vi "Safety systems data.vi"(7 "Arm System Status":bool, 8 "safety system raw data":string) -> (0 "Laser 2":bool, 1 "Safety System 2":bool[](array[boolean]), 2 "Laser 1":bool, 3 "Safety System 1":bool[](array[boolean]))   [LabVIEW 2020]
panel:
  out "number":u32
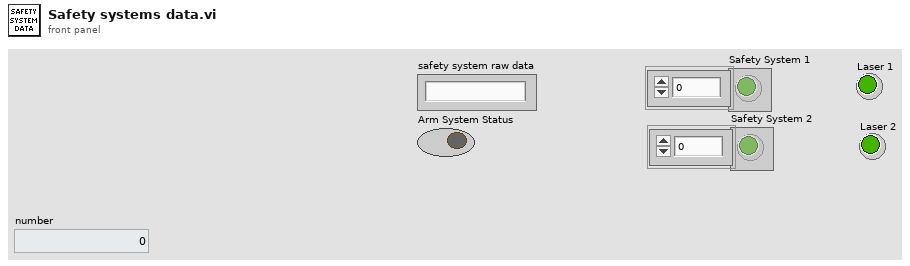
[diagram p1: front panel]
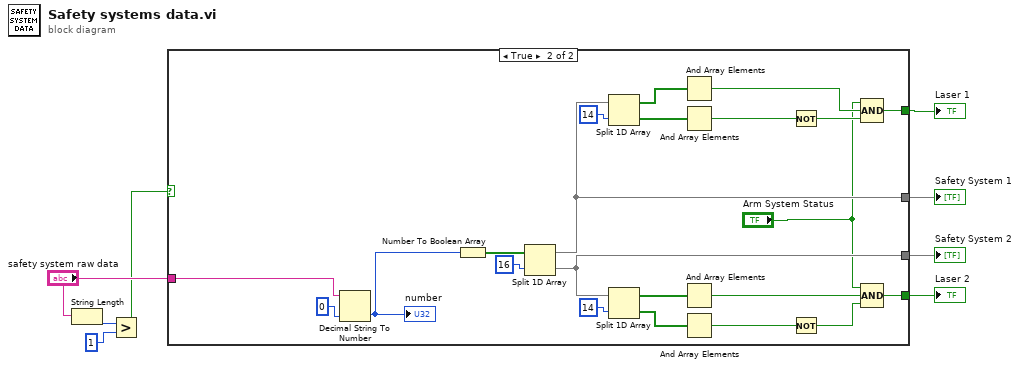
[diagram p0: block diagram]
diagram:
  n1 = String Length(string="safety system raw data") -> (length=w3:i32)
  n2 = Greater?(x=w3, y=1) -> (0:w1:bool)
  n3 = case shown="True" w1 {
    tunnel: [_ w24] -> w8
    tunnel: [_ w23] -> w7
    tunnel: [_ w11] -> w6
    tunnel: [_ w10] -> w5
    tunnel: "safety system raw data" -> [_ w9]
    frame False {
    }
    frame True {
      n4 = Decimal String To Number(string=w9, default (0L)=u32 0) -> (number=w30:u32)  [unwired: 1 in, 1 out]
      "number" <- w30
      n5 = Number To Boolean Array(number=w30) -> (Boolean array=w28:bool[])
      n6 = Split 1D Array(array=w28, index=16) -> (first subarray=w23:bool[], second subarray=w24:bool[])
      n7 = Split 1D Array(array=w23, index=14 ("length")) -> (first subarray=w22:bool[], second subarray=w17:bool[])
      n8 = Split 1D Array(array=w24, index=14 ("length")) -> (first subarray=w21:bool[], second subarray=w20:bool[])
      n9 = And Array Elements(Boolean array=w22) -> (logical AND=w15:bool)
      n10 = And Array Elements(Boolean array=w17) -> (logical AND=w18:bool)
      n11 = And Array Elements(Boolean array=w21) -> (logical AND=w13:bool)
      n12 = And Array Elements(Boolean array=w20) -> (logical AND=w19:bool)
      n13 = Not(x=w18) -> (.not. x?=w16:bool)
      n14 = Not(x=w19) -> (.not. x?=w14:bool)
      n15 = Compound Arithmetic op=AND("Arm System Status", w15, w16) -> (w11:bool)
      n16 = Compound Arithmetic op=AND("Arm System Status", w13, w14) -> (w10:bool)
    }
  }
  "Safety System 1" <- w7
  "Safety System 2" <- w8
  "Laser 1" <- w6
  "Laser 2" <- w5
